vi "CliReadSZL.vi"(0 "ref in":u64, 5 "ID":i32, 7 "Index":i32, 11 "error in (no error)":errorcluster) -> (2 "LENTHDR":u16, 3 "N_DR":u16, 4 "ref out":u64, 6 "Result":i32, 13 "Size":i32, 14 "pUsrData":u8[](array[numeric]), 15 "error out":errorcluster)   [LabVIEW 2020, in "Snap7.lvlib"]
uses:
  Snap7.lvlib
  windows/lv_snap7.dll
panel:
  in  "var Size":i32
  in  "var N_DR":u16
  in  "var LENTHDR":u16
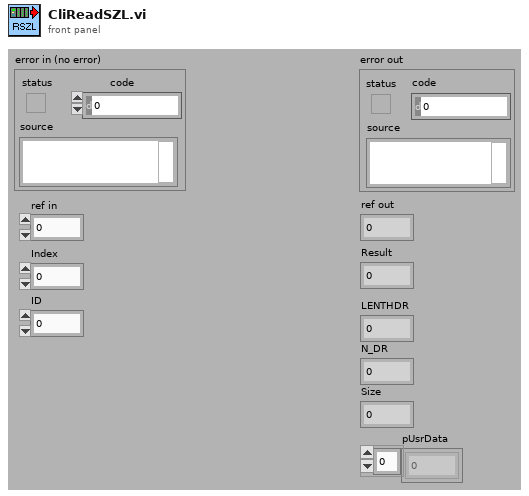
[diagram p1: front panel]
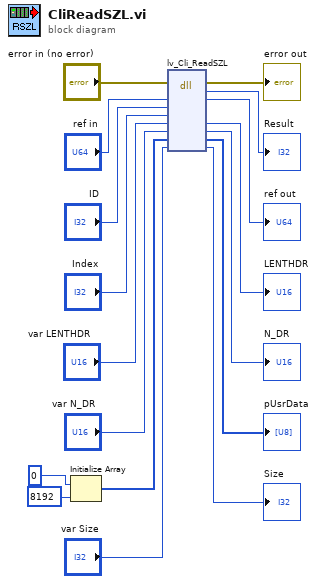
[diagram p0: block diagram]
diagram:
  n1 = Initialize Array(u8 0, 8192) -> (w8:u8[])
  n2 = dll-call lib="PTH2iabs CUsersFeng项目HLCEPS300-1老性能试验台SourcesSnap7libwindowslv_snap7.dll" fn="lv_Cli_ReadSZL"(error in="error in (no error)", "Client"="ref in", "ID"="ID", "Index"="Index", "LENTHDR"="var LENTHDR", "N_DR"="var N_DR", "pUsrData"=w8, "Size"="var Size") -> (error out=→"error out":errorcluster, "return type"=→"Result":i32, "Client"=→"ref out":u64, "LENTHDR"=→"LENTHDR":u16, "N_DR"=→"N_DR":u16, "pUsrData"=→"pUsrData":u8[], "Size"=→"Size":i32)  [unwired: 4 in, 1 out]
